vi "Vechicle Boot Sequence.vi"(0 "Simulate BMS LV":bool=TRUE, 1 "Simulate Motors":bool=TRUE, 2 "Simulate BMS":bool=TRUE, 3 "Simulate Dashboard":bool=TRUE, 4 "Don't irritate me":bool, 5 "Dashboard Control in":T1={"Tractive System"=TRUE, "RTD"=TRUE, "AMS error"=TRUE, "IMD error"=TRUE, "Low Voltage"=0.0, "High Voltage"=0.0} {"High Voltage" scale=0.0..10.0; "Low Voltage" scale=0.0..10.0}, 7 "error in":errorcluster, 10 "CAN Session":T2, 12 "CANOpen Session":refnum<k20>) -> (20 "Left motor Clustered SDO":T4, 21 "Right motor Clustered SDO":T4, 22 "Battery Status":T6, 23 "BMS Low Voltage Status":T3 {"Temp. 0" scale=0.0..80.0; "Temp. 1" scale=0.0..80.0}, 25 "Dashboard Control out":T1={"Tractive System"=TRUE, "RTD"=TRUE, "AMS error"=TRUE, "IMD error"=TRUE, "Low Voltage"=0.0, "High Voltage"=0.0} {"High Voltage" scale=0.0..10.0; "Low Voltage" scale=0.0..10.0}, 27 "error out":errorcluster)   [LabVIEW 2016]
uses:
  RT/Battery Status.ctl
  RT/Clustered SDO.ctl
  RT/BMS Voltage status 2.ctl
  Dashboard Control.ctl
  Program Files (x86)/National Instruments/LabVIEW 2016/examples/robotics/EPOS2 CANOpen Driver/Low Level VIs/Typedefs/CAN Refnum.ctl
  Program Files (x86)/National Instruments/LabVIEW 2016/examples/robotics/EPOS2 CANOpen Driver/Low Level VIs/Typedefs/CAN Session Pointer.ctl
  Program Files (x86)/National Instruments/LabVIEW 2016/examples/robotics/EPOS2 CANOpen Driver/Low Level VIs/Typedefs/CAN Communication References.ctl
  Program Files (x86)/National Instruments/LabVIEW 2016/examples/robotics/EPOS2 CANOpen Driver/Low Level VIs/Typedefs/kill process notifier array.ctl
  Program Files (x86)/National Instruments/LabVIEW 2016/examples/robotics/EPOS2 CANOpen Driver/Low Level VIs/Typedefs/Write Queue.ctl
  Program Files (x86)/National Instruments/LabVIEW 2016/examples/robotics/EPOS2 CANOpen Driver/Low Level VIs/Typedefs/FPGA CAN Frame Cluster.ctl
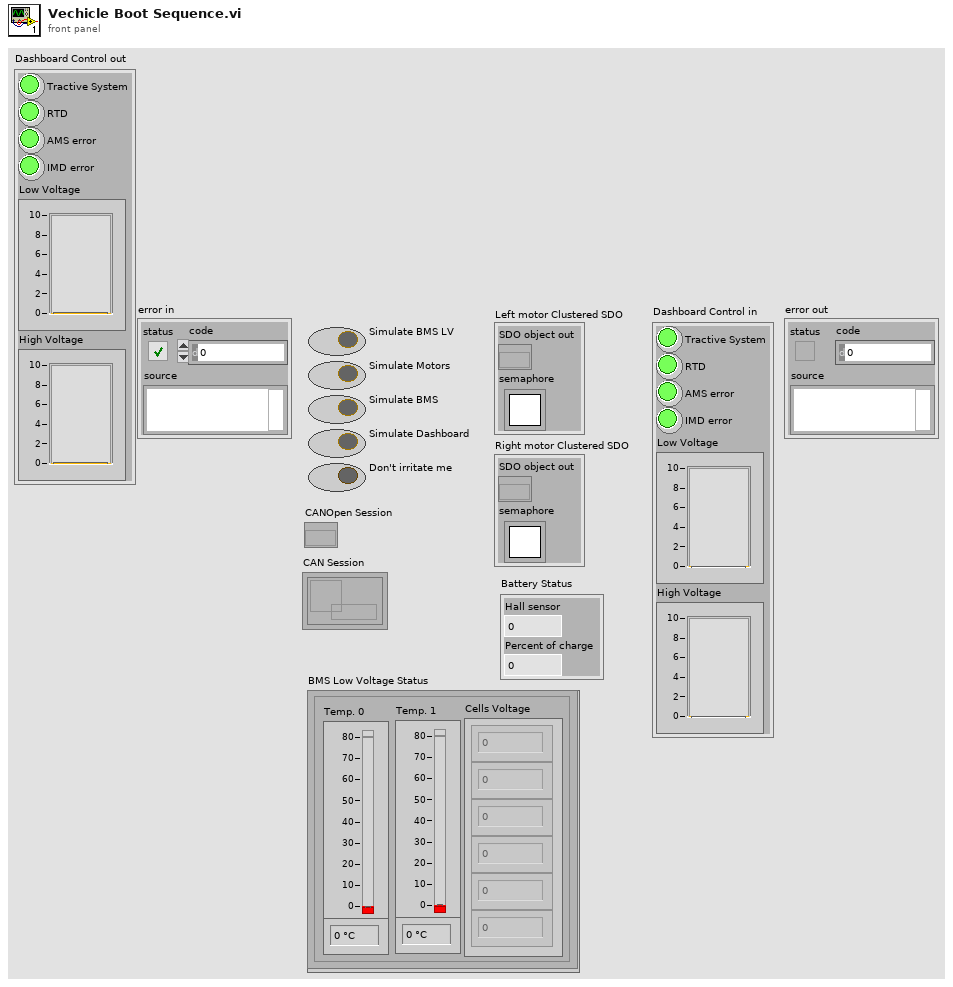
[diagram p1: front panel]
types:
  T1 = typedef "Dashboard Control.ctl" = cluster{"Tractive System":bool, "RTD":bool, "AMS error":bool, "IMD error":bool, "Low Voltage":dbl, "High Voltage":dbl}
  T2 = typedef "CAN Refnum.ctl" = refnum<k1>
  T3 = typedef "BMS Voltage status 2.ctl" = cluster{"Cells Voltage":dbl[], "Temp. 1":u8, "Temp. 0":u8}
  T4 = typedef "Clustered SDO.ctl" = cluster{"SDO object out":refnum<k20>, "semaphore":T5}
  T5 = typedef "Semaphore RefNum" = refnum<k1>
  T6 = typedef "Battery Status.ctl" = cluster{"Hall sensor":i32, "Percent of charge":i16}
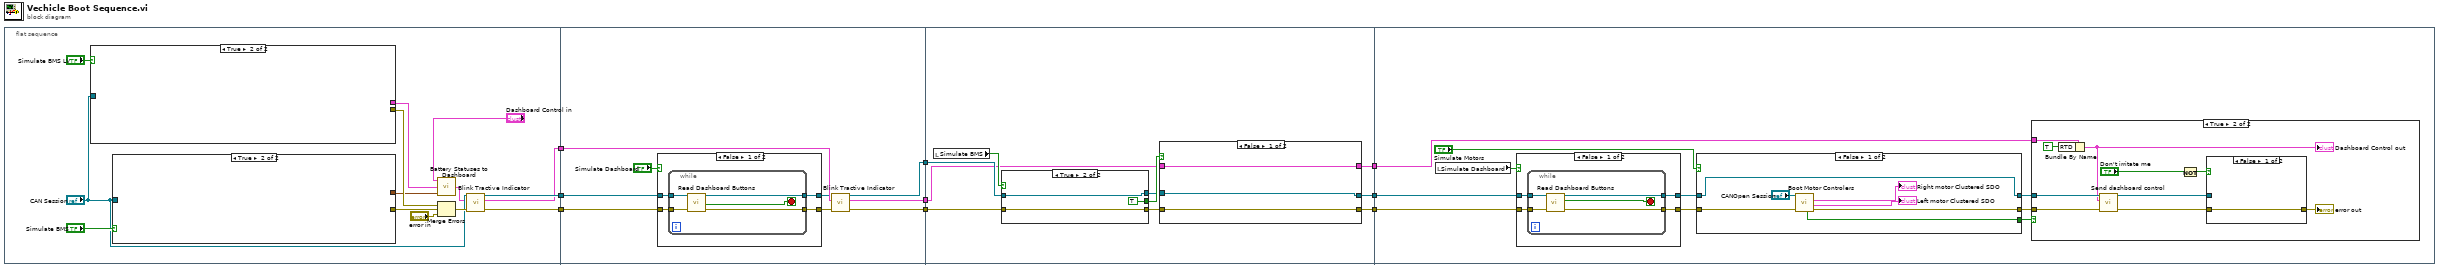
[diagram p0: block diagram]
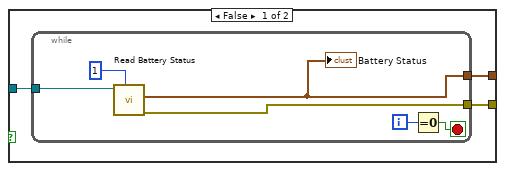
[diagram p2: hidden frame]
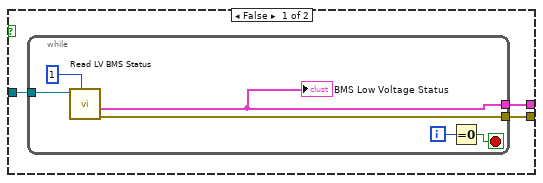
[diagram p3: hidden frame]
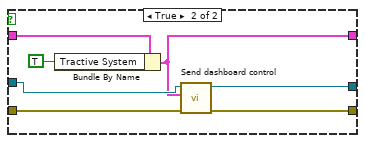
[diagram p5: hidden frame]
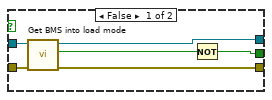
[diagram p6: hidden frame]
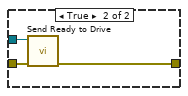
[diagram p9: hidden frame]
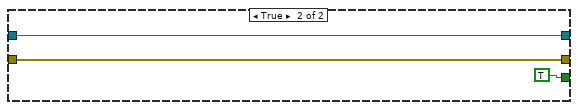
[diagram p10: hidden frame]
diagram:
  n1 = flat-sequence {
    tunnel: [w20] -> w9
    tunnel: [w19] -> w8
    tunnel: [w18] -> w7
    tunnel: w9 -> [w50]
    tunnel: w8 -> [w49]
    tunnel: w7 -> [w47]
    tunnel: [w46] -> w6
    tunnel: [w45] -> w5
    tunnel: [w44] -> w4
    tunnel: w6 -> [w70]
    tunnel: w5 -> [w69]
    tunnel: w4 -> [w65]
    tunnel: [w64] -> w3
    tunnel: [w63] -> w2
    tunnel: [w62] -> w1
    tunnel: w3 -> [w100]
    tunnel: w2 -> [w99]
    tunnel: w1 -> [w91]
    frame #0 {
      n2 = case shown="True" "Simulate BMS LV" {
        tunnel: [w35 _] -> w23
        tunnel: "CAN Session" -> [w34 _]
        tunnel: [w33 _] -> w13
        frame False {
          n3 = while {
            tunnel: [w39] -> w35
            tunnel: w34 -> [w37]
            tunnel: [w38] -> w33
            i -> [w40]
            stop <- w41 stop-if-true
            n4 = call "Read LV BMS Status.vi"("timeout in ms (-1)"=1, "CAN Session In"=w37) -> ("error out"=w39:errorcluster, "BMS Low Voltage Status"=w38:T3)  [unwired: 7 in, 1 out]
            "BMS Low Voltage Status" <- w38
            n5 = Equal To 0?(x=w40) -> (x = 0?=w41:bool)
          }
        }
        frame True {
        }
      }
      n6 = case shown="True" "Simulate BMS" {
        tunnel: [w26 _] -> w22
        tunnel: "CAN Session" -> [w25 _]
        tunnel: [w24 _] -> w12
        frame False {
          n7 = while {
            tunnel: [w30] -> w26
            tunnel: w25 -> [w29]
            tunnel: [w28] -> w24
            i -> [w31]
            stop <- w32 stop-if-true
            n8 = call "Read Battery Status.vi"("timeout in ms (-1)"=1, "CAN Session In"=w29) -> ("error out"=w30:errorcluster, "Battery Status"=w28:T6)  [unwired: 7 in, 1 out]
            "Battery Status" <- w28
            n9 = Equal To 0?(x=w31) -> (x = 0?=w32:bool)
          }
        }
        frame True {
        }
      }
      n10 = call "Battery Statuses to Dashboard.vi"("Battery Status"=w12, "BMS Low Voltage Status"=w13, "Dashboard Control in"="Dashboard Control in") -> ("Dashboard Control out"=w11:T1)
      n11 = Merge Errors(w23, w22, "error in") -> (w21:errorcluster)
      n12 = call "Blink Tractive Indicator.vi"("error in"=w21, "Dashboard Control in"=w11, "CAN Session In"="CAN Session") -> ("error out"=w20:errorcluster, "Dashboard Control out"=w18:T1, "CAN Session Out"=w19:T2)  [unwired: 6 in]
    }
    frame #1 {
      n13 = case shown="False" "Simulate Dashboard" {
        tunnel: w50 -> [w54 w61]
        tunnel: w49 -> [w53 w60]
        tunnel: [w52 w61] -> w48
        tunnel: [w51 w60] -> w43
        frame False {
          n14 = while {
            tunnel: w54 -> [w59]
            tunnel: w53 -> [w58]
            tunnel: [w57] -> w52
            tunnel: [w55] -> w51
            stop <- w56 stop-if-true
            n15 = call "Read Dashboard Buttons.vi"("error in"=w59, "CAN Session In"=w58) -> ("error out"=w57:errorcluster, "Tractive system activation"=w56:bool, "CAN Session Out"=w55:T2)  [unwired: 6 in, 1 out]
          }
        }
        frame True {
        }
      }
      n16 = call "Blink Tractive Indicator.vi"("error in"=w48, "Dashboard Control in"=w47, "CAN Session In"=w43) -> ("error out"=w45:errorcluster, "Dashboard Control out"=w44:T1, "CAN Session Out"=w46:T2)  [unwired: 6 in]
    }
    frame #2 {
      n17 = local read "Simulate BMS"() -> (w71:bool)
      n18 = case shown="True" w71 {
        tunnel: w69 -> [w87 w90]
        tunnel: [w86 w90] -> w67
        tunnel: w70 -> [w84 w88]
        tunnel: [w83 TRUE] -> w68
        tunnel: [w82 w88] -> w66
        frame False {
          n19 = call "Get BMS into load mode.vi"("error in"=w87, "CAN Session In"=w84) -> ("error out"=w86:errorcluster, "Error"=w85:bool, "CAN Session Out"=w82:T2)  [unwired: 7 in]
          n20 = Not(x=w85) -> (.not. x?=w83:bool)
        }
        frame True {
        }
      }
      n21 = case shown="False" w68 {
        tunnel: w67 -> [w74 w81]
        tunnel: w66 -> [w73 w80]
        tunnel: w65 -> [w72 w78]
        tunnel: [w74 w77] -> w64
        tunnel: [w73 w76] -> w63
        tunnel: [w72 w75] -> w62
        frame False {
        }
        frame True {
          n22 = Bundle By Name(cluster=w78, "Tractive System"=TRUE) -> (w75:T1)
          n23 = call "Send dashboard control.vi"("error in"=w81, "Dashboard Control"=w75, "CAN Session In"=w80) -> ("error out"=w77:errorcluster, "CAN Session Out"=w76:T2)  [unwired: 7 in]
        }
      }
    }
    frame #3 {
      n24 = local read "Simulate Dashboard"() -> (w93:bool)
      n25 = case shown="False" w93 {
        tunnel: w100 -> [w104 w110]
        tunnel: w99 -> [w103 w111]
        tunnel: [w102 w110] -> w98
        tunnel: [w101 w111] -> w95
        frame False {
          n26 = while {
            tunnel: w104 -> [w109]
            tunnel: w103 -> [w108]
            tunnel: [w106] -> w102
            tunnel: [w107] -> w101
            stop <- w105 stop-if-true
            n27 = call "Read Dashboard Buttons.vi"("error in"=w109, "CAN Session In"=w108) -> ("error out"=w106:errorcluster, "Ready to drive"=w105:bool, "CAN Session Out"=w107:T2)  [unwired: 6 in, 1 out]
          }
        }
        frame True {
        }
      }
      n28 = case shown="False" "Simulate Motors" {
        tunnel: [w130 w134] -> w96
        tunnel: [w129 TRUE] -> w97
        tunnel: w98 -> [w128 w134]
        tunnel: w95 -> [w127 w133]
        tunnel: [w127 w133] -> w94
        frame False {
          n29 = call "Boot Motor Controlers.vi"("error in (no error)"=w128, "CANOpen Session in"="CANOpen Session") -> ("error out"=w130:errorcluster, "Left motor Clustered SDO"=→"Left motor Clustered SDO":T4, "Right motor Clustered SDO"=→"Right motor Clustered SDO":T4, "Error"=w129:bool)  [unwired: 5 in, 1 out]
        }
        frame True {
        }
      }
      n30 = case shown="True" w97 {
        tunnel: w94 -> [_ w117]
        tunnel: w96 -> [_ w118]
        tunnel: w91 -> [_ w116]
        frame False {
        }
        frame True {
          n31 = Bundle By Name(cluster=w116, "RTD"=TRUE) -> (w114:T1)
          "Dashboard Control out" <- w114
          n32 = call "Send dashboard control.vi"("error in"=w118, "Dashboard Control"=w114, "CAN Session In"=w117) -> ("error out"=w119:errorcluster, "CAN Session Out"=w120:T2)  [unwired: 7 in]
          n33 = Not(x="Don't irritate me") -> (.not. x?=w112:bool)
          n34 = case shown="False" w112 {
            tunnel: [w122 w125] -> w121
            tunnel: w120 -> [_ w124]
            tunnel: w119 -> [w122 w123]
            frame False {
            }
            frame True {
              n35 = call "Send Ready to Drive.vi"("error in"=w123, "CAN Session In"=w124) -> ("error out"=w125:errorcluster)  [unwired: 8 in, 1 out]
            }
          }
          "error out" <- w121
        }
      }
    }
  }
